vi "Search Document Bench.vi"(8 "entrée d'erreur (pas d'erreur)":errorcluster, 11 "Firebase Altyor en entrée":refnum<class "Firebase Altyor.lvclass">) -> (0 "sortie d'erreur":errorcluster, 2 "Source":string, 3 "Firebase Altyor en sortie":refnum<class "Firebase Altyor.lvclass">)   [LabVIEW 2020, in "Library Instrument & Equipement.lvlib" / "Library FireBase.lvlib" / "Firebase Altyor.lvclass"]
uses:
  Firebase Altyor.lvclass
  C:/Users/ngarcin/OneDrive - Altyor/Standard TB/Class/Firebase/Source/Firebase Driver/Firebase Driver.lvclass
  Commun VI/TypeDef/Liste Error.ctl
  Firebase Altyor.lvclass/Firebase Altyor.ctl
  Commun VI/Library Commun.lvlib
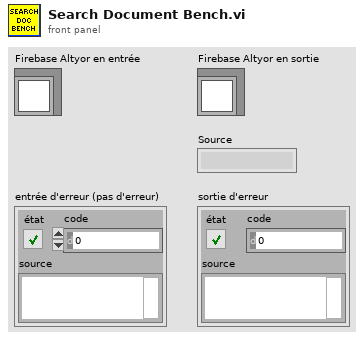
[diagram p1: front panel]
types:
  T1 = typedef "Library Commun.lvlib/Liste Error.ctl" = enum16{"Firebase Driver - Get Document", "Firebase Driver - Get Document With Where", "Firebase Driver - Delete Document", "Firebase Driver - Set Document", "Firebase Driver - Update Document", "Firebase Altyor - Search Document Bench", "Firebase Altyor - Class Not in Firebase", "Spectrum_Analyser - Timeout", "Relay Board - Qty Relay", "DIO - Pb Funtion", "Power_Supply - Peripherical not find", "Mutimeter - Peripherical not find", "Instrument - Function Not Used", "Instrument - Instrument name not specified", "Instrument - Allready Initialised", "Instrument - TimeOut", "Instrument - the instrument must be Initialise before", "Instrument - Frame Not received", "Instrument - Frame Nok", "Test - Initialise the File_for_Save", "Test - Timeout", "Test - Cmd Error", "FGV - Variable ", "BDD FireBase - Define Class", "SN - Class Not Define"}
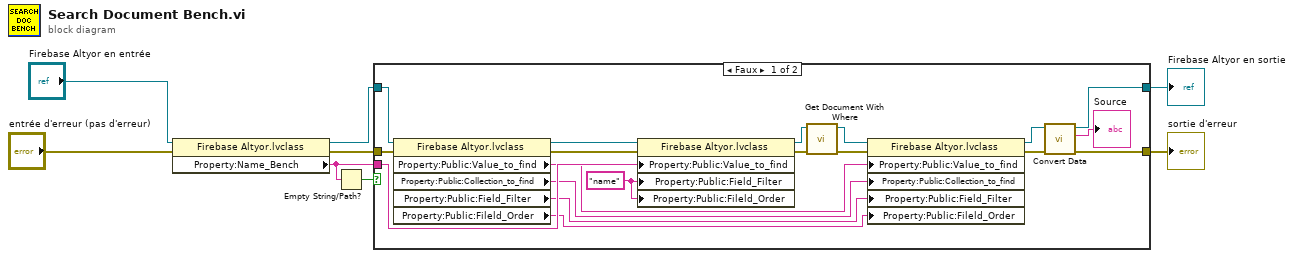
[diagram p0: block diagram]
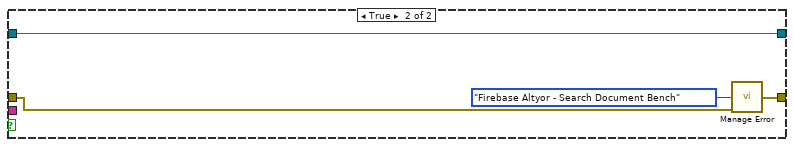
[diagram p2: hidden frame]
diagram:
  n1 = property class="Firebase Altyor.lvclass"(reference="Firebase Altyor en entrée", error in="entrée d'erreur (pas d'erreur)") -> (reference out=w1:refnum<class "Firebase Altyor.lvclass">, error out=w4:errorcluster, "Property:Name_Bench"=w3:string)
  n2 = Empty String/Path?(string/path=w3) -> (empty?=w6:bool)
  n3 = case shown="Faux" w6 {
    tunnel: [w24 w29] -> w8
    tunnel: w4 -> [w22 w28]
    tunnel: w1 -> [w20 w31]
    tunnel: w3 -> [w14 _]
    tunnel: [w19 w31] -> w7
    frame False {
      w12 = "name" ("Field_Filter")
      n4 = property class="Firebase Altyor.lvclass"(reference=w20, error in=w22) -> (reference out=w23:refnum<class "Firebase Altyor.lvclass">, error out=w21:errorcluster, "Property:Public:Value_to_find"=w13:string, "Property:Public:Collection_to_find"=w11:string, "Property:Public:Field_Filter"=w10:string, "Property:Public:Fileld_Order"=w9:string)
      n5 = property class="Firebase Altyor.lvclass"(reference=w23, error in=w21, "Property:Public:Value_to_find"=w14, "Property:Public:Field_Filter"=w12, "Property:Public:Fileld_Order"=w12) -> (reference out=w26:refnum<class "Firebase Altyor.lvclass">, error out=w27:errorcluster)
      n6 = call-dynamic "Get Document With Where.vi"("error in (no error)"=w27, "Firebase (Default) en entrée"=w26) -> ("error out"=w18:errorcluster, "Firebase (Default) en sortie"=w16:refnum<class "Firebase Altyor.lvclass">)  [unwired: 8 in]
      n7 = property class="Firebase Altyor.lvclass"(reference=w16, error in=w18, "Property:Public:Value_to_find"=w13, "Property:Public:Collection_to_find"=w11, "Property:Public:Field_Filter"=w10, "Property:Public:Fileld_Order"=w9) -> (reference out=w15:refnum<class "Firebase Altyor.lvclass">, error out=w17:errorcluster)
      n8 = call "Convert Data.vi"("entrée d'erreur (pas d'erreur)"=w17, "Firebase Altyor en entrée"=w15) -> ("sortie d'erreur"=w24:errorcluster, "Source"=→"Source":string, "Firebase Altyor en sortie"=w19:refnum<class "Firebase Altyor.lvclass">)  [unwired: 6 in, 1 out]
    }
    frame True {
      n9 = call "Manage Error.vi"("Code Erreur"=Liste_Error."Firebase Altyor - Search Document Bench", "error in (no error)"=w28) -> ("error out"=w29:errorcluster)  [unwired: 13 in]
    }
  }
  "sortie d'erreur" <- w8
  "Firebase Altyor en sortie" <- w7
